vi "getMessage.vi"(8 "error in (no error)":errorcluster, 11 "Instance In":refnum<data-value>) -> (0 "error out":errorcluster, 2 "Message":string, 3 "Instance out":refnum<data-value>)   [LabVIEW 2017, in "SingleObject.lvclass"]
uses:
  SingleObject.lvclass
  SingleObject.lvclass/SingleObject.ctl
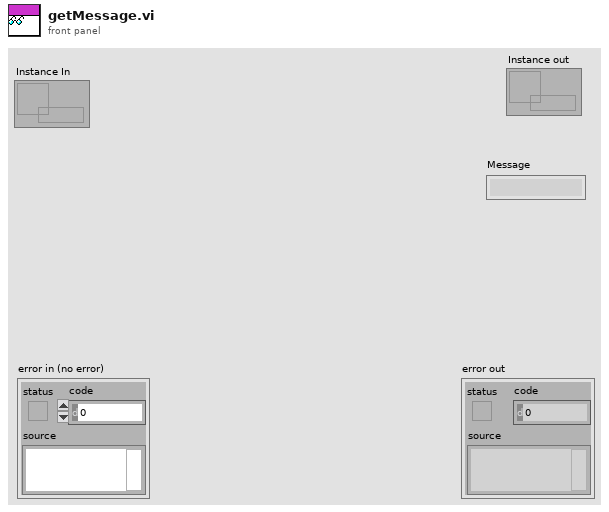
[diagram p1: front panel]
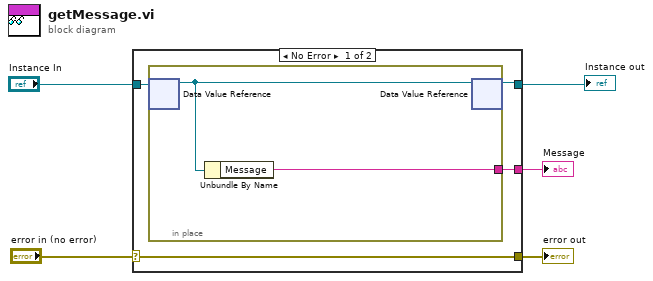
[diagram p0: block diagram]
diagram:
  n1 = case shown="No Error" "error in (no error)" {
    selector: "error in (no error)" -> [w9 w12]
    tunnel: [w9 w12] -> w4
    tunnel: [w6 w13] -> w1
    tunnel: "Instance In" -> [w7 w13]
    tunnel: [w8 _] -> w3
    frame No Error {
      n2 = in-place {
        in-place-border: [w11] -> w8
        n3 = in-place-dvr #1(w7) -> (w10:refnum<class "SingleObject.lvclass">)  [unwired: 1 out]
        n4 = Unbundle By Name(w10) -> ("Message"=w11:string)
        n5 = in-place-dvr #1(w10) -> (w6:refnum<data-value>)  [unwired: 1 out]
      }
    }
    frame Error {
    }
  }
  "error out" <- w4
  "Message" <- w3
  "Instance out" <- w1
